vi "Test_InsertCount.vi"(8 "error in (no error)":errorcluster, 11 "TestCase in":refnum<class "ListImp_Functional.lvclass">) -> (0 "error out":errorcluster, 3 "TestCase out":refnum<class "ListImp_Functional.lvclass">)   [LabVIEW 2009, in "ListImp_Functional.lvclass"]
uses:
  ListImp_Functional.lvclass
  ListImp_Functional.lvclass/ListImp_Functional.ctl
  source/Lists/List/List.lvclass
  source/Lists.Interfaces/String/String.lvclass
  UnitTestComparisons/UnitTestComparisons.lvlib
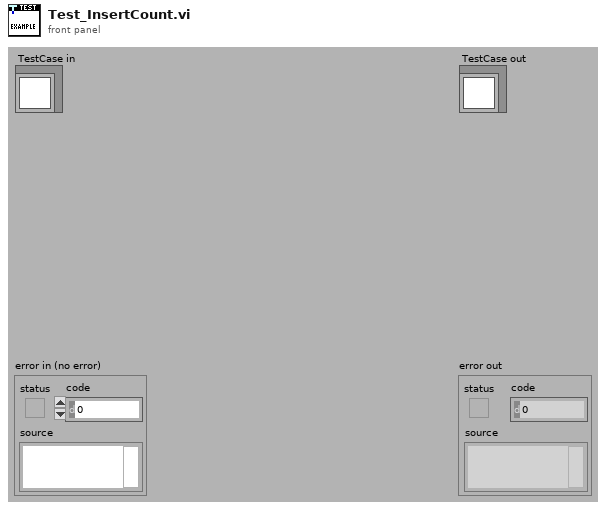
[diagram p1: front panel]
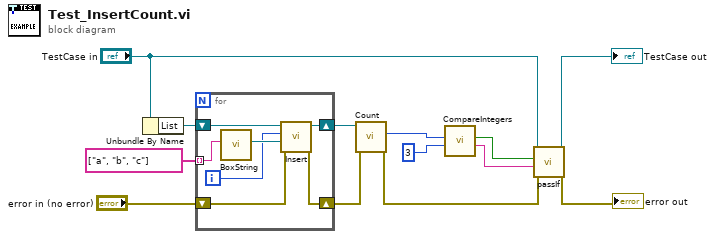
[diagram p0: block diagram]
diagram:
  n1 = Unbundle By Name("TestCase in") -> ("List"=w9:refnum<class "List.lvclass">)
  n2 = for {
    tunnel: string[] ["a", "b", "c"] -> [w17] mode=indexing
    shift-right: [w19] -> w7
    shift-left: w9 -> [w20]
    shift-right: [w14] -> w5
    shift-left: "error in (no error)" -> [w15]
    i -> [w16]
    n3 = call "BoxString.vi"("String"=w17) -> ("String out"=w18:refnum<class "String.lvclass">)  [unwired: 10 in]
    n4 = call-dynamic "Insert.vi"("error in (no error)"=w15, "Item"=w18, "Index"=w16, "List in"=w20) -> ("error out"=w14:errorcluster, "List out"=w19:refnum<class "List.lvclass">)  [unwired: 6 in]
  }
  n5 = call-dynamic "Count.vi"("error in (no error)"=w5, "List in"=w7) -> ("error out"=w10:errorcluster, "Number of Items"=w4:i32)  [unwired: 7 in, 1 out]
  n6 = call "CompareIntegers.vi"("Expected Value"=3 ("x"), "Actual Value"=w4) -> ("Message"=w1:string, "Equal?"=w2:bool)  [unwired: 8 in]
  n7 = call-dynamic "passIf.vi"("error in (no error)"=w10, "message (\"\")"=w1, "pass"=w2, "TestCase in"="TestCase in") -> ("error out"=→"error out":errorcluster, "TestCase out"=→"TestCase out":refnum<class "ListImp_Functional.lvclass">)  [unwired: 6 in]
